vi "EncoderAveragingTool.vi"(8 "Avg Size":dbl, 10 "Reading":dbl, 11 "Array":dbl[](array[numeric])) -> (2 "Avg Val":dbl, 3 "Array 2":dbl[](array[numeric]))   [LabVIEW 2016]
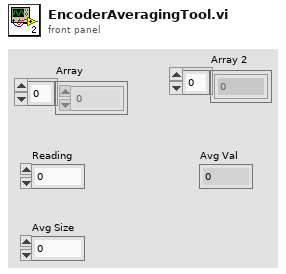
[diagram p1: front panel]
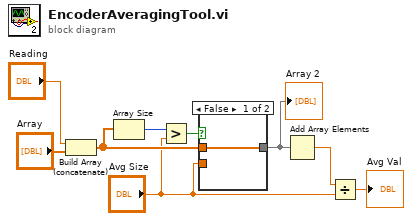
[diagram p0: block diagram]
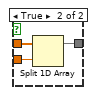
[diagram p2: hidden frame]
diagram:
  n1 = Build Array (concatenate)("Reading", "Array") -> (w5:dbl[])
  n2 = Array Size(array=w5) -> (size(s)=w7:i32)
  n3 = Greater?(x=w7, y="Avg Size") -> (0:w6:bool)
  n4 = case shown="False" w6 {
    tunnel: w5 -> [w10 w13]
    tunnel: "Avg Size" -> [_ w12]
    tunnel: [w10 w11] -> w4
    frame False {
    }
    frame True {
      n5 = Split 1D Array(array=w13, index=w12) -> (first subarray=w11:dbl[])  [unwired: 1 out]
    }
  }
  "Array 2" <- w4
  n6 = Add Array Elements(numeric array=w4) -> (sum=w3:dbl)
  n7 = Divide(x=w3, y="Avg Size") -> (x/y=→"Avg Val":dbl)
